vi "ActionVIOnLoad.Section.Move.vi"(7 "Type":T2, 8 "error in (no error)":errorcluster, 9 "Paste Parent GUID":string, 10 "Copy Parent GUID":string, 11 "Section Ref in":T1 format="%.0x") -> (0 "error out":errorcluster, 3 "Section Ref out":T1 format="%.0x")   [LabVIEW 2015, in "Diagnostics Addon System Explorer.lvlib"]
uses:
  Diagnostics Addon System Explorer.lvlib
  Shared/Types/Type.ctl
  <vilib>/NI Veristand/Custom Device API/Custom Device Item Ref.ctl
  Types/Frame.Export.ctl
  Shared/Types/Signal.ctl
  <vilib>/NI Veristand/Custom Device Tools/Custom Device Utility Library/NI VeriStand - Search for Item by GUID.vi
  <vilib>/NI Veristand/Custom Device API/Get Item Property (Variant).vi
  <vilib>/NI Veristand/Custom Device Tools/Custom Device Utility Library/Custom Device Utility Library.lvlib
  Shared/Diagnostics Addon Shared.lvlib
  <vilib>/NI Veristand/Custom Device API/Custom Device API.lvlib
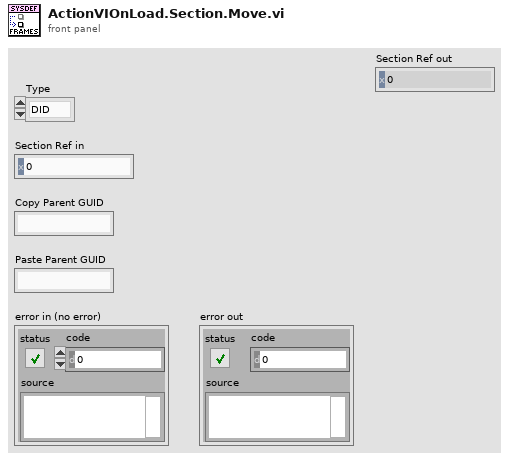
[diagram p1: front panel]
types:
  T1 = typedef "Custom Device API.lvlib/Custom Device Item Ref.ctl" = u64
  T2 = typedef "Diagnostics Addon Shared.lvlib/Type.ctl" = enum16{"DID", "CDID", "PID", "CPID", "Read Memory", "Write Memory", "DTC Control", "IO Cmd", "IO Resp", "Routine Start Cmd", "Routine Start Resp", "Routine Request Cmd", "Routine Request Resp", "Routine Stop Cmd", "Routine Stop Resp"}
  T3 = typedef "Diagnostics Addon System Explorer.lvlib/Frame.Export.ctl" = cluster{"Name":string, "Description":string, "ID":u32, "Signals":T4[]}
  T4 = typedef "Diagnostics Addon Shared.lvlib/Signal.ctl" = cluster{"Start Bit":u8, "Length":u8, "Scaling Factor":dbl, "Scaling Offset":dbl, "Minimum":dbl, "Maximum":dbl, "Data Type":u32, "Byte Order":u32, "Default Value":dbl, "Name":string, "Units":string, "Description":string}
  T5 = typedef "Custom Device API.lvlib/Custom Device Item Info.ctl" = cluster{"Name":string, "Is Channel":bool, "GUID":string, "Is Waveform":bool}
  T6 = cluster{"Start Bit":u8, "Length":u8, "Scaling Factor":dbl, "Scaling Offset":dbl, "Minimum":dbl, "Maximum":dbl, "Data Type":u32, "Byte Order":u32, "Default Value":dbl, "Name":string, "Units":string, "Description":string}
  T7 = typedef "Custom Device API.lvlib/Custom Device Channel.ctl" = cluster{"Type":T8, "Units":string, "Default Value":dbl, "Faultable":bool, "Scalable":bool}
  T8 = typedef "Custom Device API.lvlib/Custom Device Channel Type.ctl" = enum16{"Input", "Output"}
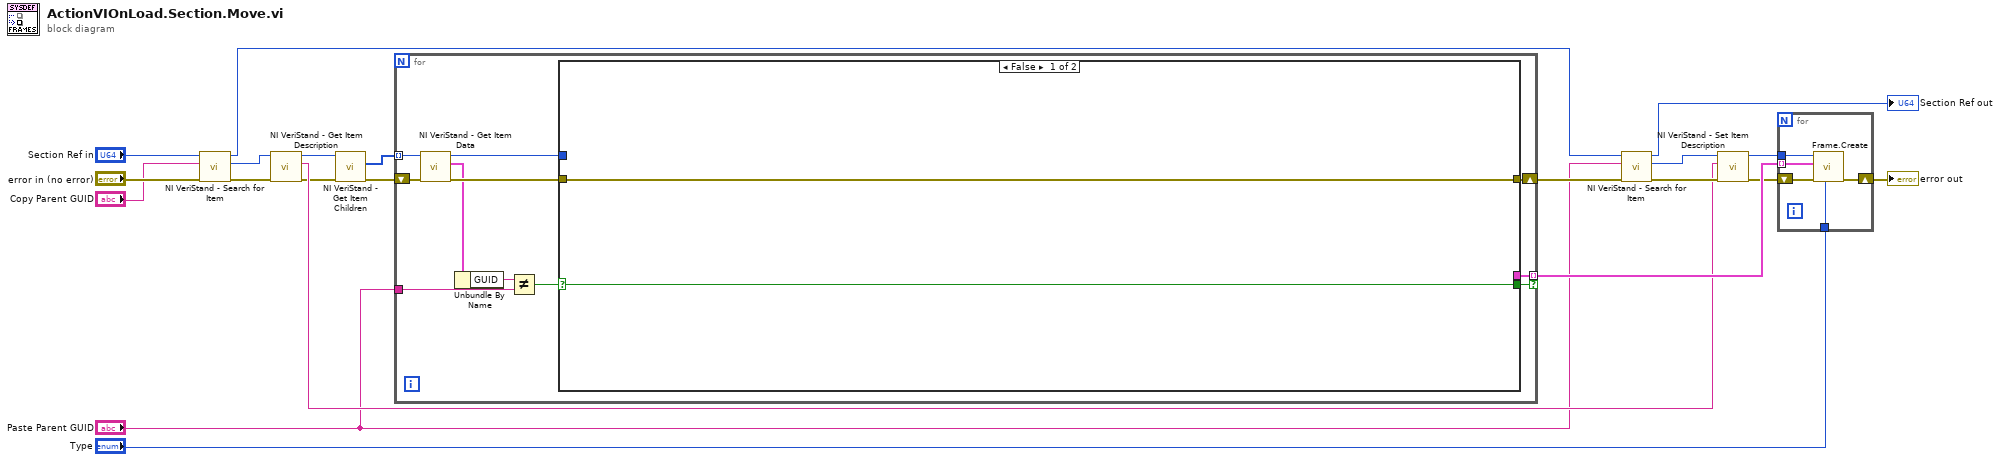
[diagram p0: block diagram]
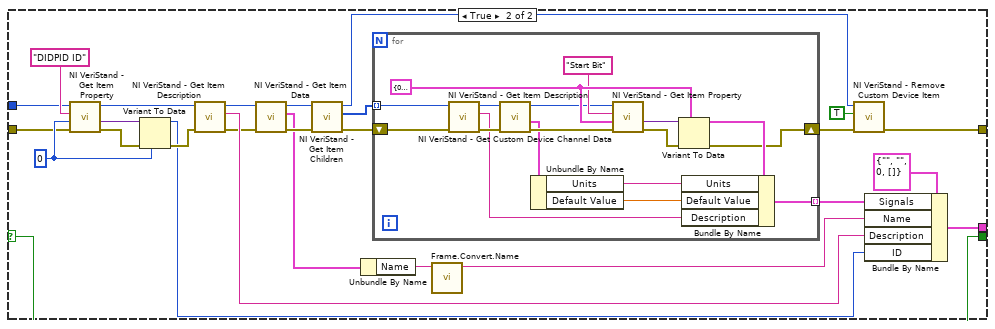
[diagram p2: hidden frame]
diagram:
  n1 = call-poly <vilib>:"NI VeriStand - Search for Item.vi"("error in"="error in (no error)", "Item GUID"="Copy Parent GUID", "Section Ref in"="Section Ref in") -> ("error out"=w10:errorcluster, "Item Ref"=w11:T1, "Section Ref out"=w18:T1)  [unwired: 5 in, 1 out]
  n2 = call <vilib>:"NI VeriStand - Get Item Description.vi"("error in (no error)"=w10, "Item Ref in"=w11) -> ("error out"=w5:errorcluster, "Description"=w12:string, "Item Ref out"=w20:T1)  [unwired: 6 in, 1 out]
  n3 = call <vilib>:"NI VeriStand - Get Item Children.vi"("error in (no error)"=w5, "Item Ref in"=w20) -> ("error out"=w4:errorcluster, "Child Refs"=w21:T1[])  [unwired: 6 in, 2 out]
  n4 = for {
    shift-right: [w31] -> w2
    shift-left: w4 -> [w30]
    tunnel: w21 -> [w28] mode=indexing
    tunnel: [w32] -> w13 mode=indexing if=w22
    tunnel: "Paste Parent GUID" -> [w24]
    n5 = call <vilib>:"NI VeriStand - Get Item Data.vi"("error in (no error)"=w30, "Item Ref in"=w28) -> ("error out"=w29:errorcluster, "Item Info"=w26:T5, "Item Ref out"=w27:T1)  [unwired: 6 in, 1 out]
    n6 = Unbundle By Name(w26) -> ("GUID"=w25:string)
    n7 = Not Equal?(x=w25, y=w24) -> (x != y?=w23:bool)
    n8 = case shown="False" w23 {
      selector: w23 -> [w33 w35]
      tunnel: [_ w42] -> w32
      tunnel: [w34 w40] -> w31
      tunnel: w29 -> [w34 w37]
      tunnel: w27 -> [_ w36]
      tunnel: [w33 w35] -> w22
      frame False {
      }
      frame True {
        w61 = u16 0 ("ID")
        n9 = call-poly <vilib>:"NI VeriStand - Get Item Property.vi"("error in (no error)"=w37, "Default Value"=w61, "Property Name"="DIDPID ID" ("DIDPID_ID"), "Item Ref in"=w36) -> ("error out"=w60:errorcluster, "Value"=w59:variant, "Item Ref out"=w56:T1)  [unwired: 4 in, 1 out]
        n10 = Variant To Data(error in=w60, type=w61, Variant=w59) -> (data=w51:u16, error out=w57:errorcluster)
        n11 = call <vilib>:"NI VeriStand - Get Item Description.vi"("error in (no error)"=w57, "Item Ref in"=w56) -> ("error out"=w47:errorcluster, "Description"=w50:string, "Item Ref out"=w49:T1)  [unwired: 6 in, 1 out]
        n12 = call <vilib>:"NI VeriStand - Get Item Data.vi"("error in (no error)"=w47, "Item Ref in"=w49) -> ("error out"=w48:errorcluster, "Item Info"=w45:T5, "Item Ref out"=w46:T1)  [unwired: 6 in, 1 out]
        n13 = call <vilib>:"NI VeriStand - Get Item Children.vi"("error in (no error)"=w48, "Item Ref in"=w46) -> ("error out"=w55:errorcluster, "Child Refs"=w54:T1[], "Item Ref out"=w39:T1)  [unwired: 6 in, 1 out]
        n14 = Unbundle By Name(w45) -> ("Name"=w44:string)
        n15 = for {
          tunnel: w54 -> [w62] mode=indexing
          shift-right: [w64] -> w41
          shift-left: w55 -> [w63]
          tunnel: [w65] -> w52 mode=indexing
          w76 = T6 {"Start Bit"=0, "Length"=0, "Scaling Factor"=0.0, "Scaling Offset"=0.0, "Minimum"=0.0, "Maximum"=0.0, "Data Type"=0, "Byte Order"=0, "Default Value"=0.0, "Name"="", "Units"="", "Description"=""} ("Signal Parameters")
          n16 = call <vilib>:"NI VeriStand - Get Item Description.vi"("error in (no error)"=w63, "Item Ref in"=w62) -> ("error out"=w72:errorcluster, "Description"=w66:string, "Item Ref out"=w74:T1)  [unwired: 6 in, 1 out]
          n17 = call <vilib>:"NI VeriStand - Get Custom Device Channel Data.vi"("error in (no error)"=w72, "Channel Ref in"=w74) -> ("error out"=w71:errorcluster, "Channel"=w70:T7, "Channel Ref out"=w73:T1)  [unwired: 4 in, 3 out]
          n18 = Unbundle By Name(w70) -> ("Units"=w68:string, "Default Value"=w67:dbl)
          n19 = call-poly <vilib>:"NI VeriStand - Get Item Property.vi"("error in (no error)"=w71, "Default Value"=w76, "Property Name"="Start Bit" ("DIDPID Signal Parameters"), "Item Ref in"=w73) -> ("error out"=w78:errorcluster, "Value"=w77:variant)  [unwired: 4 in, 2 out]
          n20 = Variant To Data(error in=w78, type=w76, Variant=w77) -> (data=w69:T6, error out=w64:errorcluster)
          n21 = Bundle By Name(cluster=w69, "Units"=w68, "Default Value"=w67, "Description"=w66) -> (w65:T6)
        }
        n22 = call "Frame.Convert.Name.vi"("VS Frame Name"=w44) -> ("Frame Name"=w43:string)  [unwired: 9 in, 1 out]
        n23 = call <vilib>:"NI VeriStand - Remove Custom Device Item.vi"("error in (no error)"=w41, "Force Delete (F)"=TRUE, "Item Ref in"=w39) -> ("error out"=w40:errorcluster)  [unwired: 7 in, 1 out]
        n24 = Bundle By Name(cluster=T3 {"Name"="", "Description"="", "ID"=0, "Signals"=[]} ("Frame"), "Signals"=w52, "Name"=w43, "Description"=w50, "ID"=w51) -> (w42:T3)
      }
    }
  }
  n25 = call-poly <vilib>:"NI VeriStand - Search for Item.vi"("error in"=w2, "Item GUID"="Paste Parent GUID", "Section Ref in"=w18) -> ("error out"=w16:errorcluster, "Item Ref"=w17:T1, "Section Ref out"=→"Section Ref out":T1)  [unwired: 5 in, 1 out]
  n26 = call <vilib>:"NI VeriStand - Set Item Description.vi"("error in (no error)"=w16, "Description"=w12, "Item Ref in"=w17) -> ("error out"=w9:errorcluster, "Item Ref out"=w8:T1)  [unwired: 6 in, 1 out]
  n27 = for {
    tunnel: w8 -> [w81]
    shift-right: [w80] -> w3
    shift-left: w9 -> [w83]
    tunnel: w13 -> [w82] mode=indexing
    tunnel: "Type" -> [w79]
    n28 = call "Frame.Create.vi"("Type"=w79, "error in (no error)"=w83, "Frame"=w82, "Section Ptr"=w81) -> ("error out"=w80:errorcluster)  [unwired: 6 in, 1 out]
  }
  "error out" <- w3
